vi "RearrangeFrameByNames__slk_mt.vi"(8 "error in (no error)":errorcluster, 10 "frame names":string[](array[string]), 11 "case model in":refnum<class "CaseModel__slk_mt.lvclass">) -> (0 "error out":errorcluster, 3 "case model out":refnum<class "CaseModel__slk_mt.lvclass">)   [LabVIEW 2012, in "Lazyboots Menu Tool.lvlib" / "CaseModel__slk_mt.lvclass"]
doc: "Rearranges frame by specified names array."
uses:
  CaseModel__slk_mt.lvclass
panel:
  # "RearrangeFrameByNames__slk_mt.vi\nRearranges frame by specified names array.\n\nNOTICE -- YOU MUST LEAVE THIS NOTICE IN PLACE.\n\nCopyright (c) 2011, LIANG LIU Shawn.Liu.cn@gmail.com\nAll rights reserved.\n\nRedistribution and use in source and binary forms, with or without modification, are permitted provided that the following conditions are met:\n-Redistributions of source code must retain the above copyright notice, this list of conditions and the following disclaimer.\n-Redistributions in binary form must reproduce the above copyright notice, this list of conditions and the following disclaimer in the documentation and/or other materials provided with the distribution.\n-Neither the name of the eLp nor the names of its contributors may be used to endorse or promote products derived from this software without specific prior written permission.\n\nTHIS SOFTWARE IS PROVIDED BY THE COPYRIGHT HOLDERS AND CONTRIBUTORS \"AS IS\" AND ANY EXPRESS OR IMPLIED WARRANTIES, INCLUDING, BUT NOT LIMITED TO, THE IMPLIED WARRANTIES OF MERCHANTABILITY AND FITNESS FOR A PARTICULAR PURPOSE ARE DISCLAIMED. IN NO EVENT SHALL THE COPYRIGHT HOLDER OR CONTRIBUTORS BE LIABLE FOR ANY DIRECT, INDIRECT, INCIDENTAL, SPECIAL, EXEMPLARY, OR CONSEQUENTIAL DAMAGES (INCLUDING, BUT NOT LIMITED TO, PROCUREMENT OF SUBSTITUTE GOODS OR SERVICES; LOSS OF USE, DATA, OR PROFITS; OR BUSINESS INTERRUPTION) HOWEVER CAUSED AND ON ANY THEORY OF LIABILITY, WHETHER IN CONTRACT, STRICT LIABILITY, OR TORT (INCLUDING NEGLIGENCE OR OTHERWISE) ARISING IN ANY WAY OUT OF THE USE OF THIS SOFTWARE, EVEN IF ADVISED OF THE POSSIBILITY OF SUCH DAMAGE."
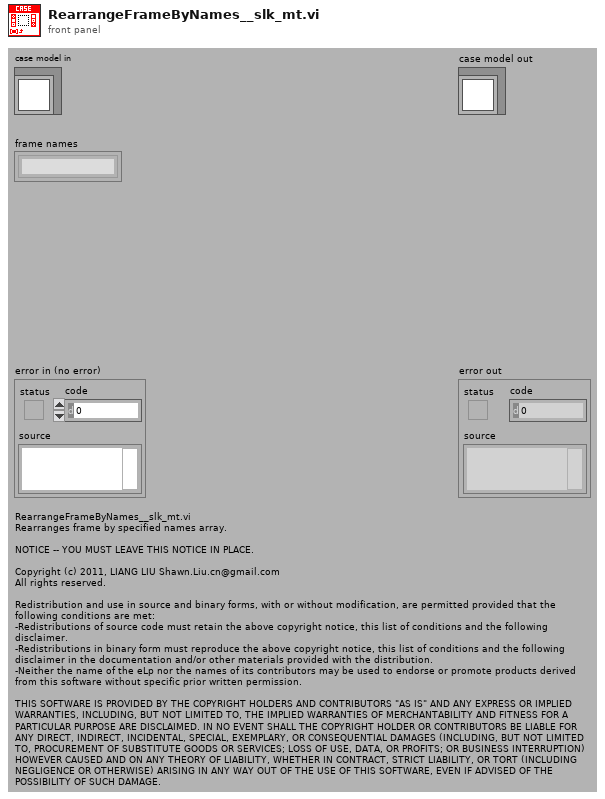
[diagram p1: front panel]
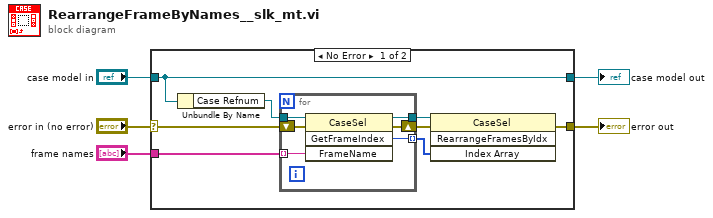
[diagram p0: block diagram]
diagram:
  n1 = case shown="No Error" "error in (no error)" {
    selector: "error in (no error)" -> [w6 w21]
    tunnel: [w9 w21] -> w4
    tunnel: [w8 w20] -> w2
    tunnel: "case model in" -> [w8 w20]
    tunnel: "frame names" -> [w7 _]
    frame No Error {
      n2 = Unbundle By Name(w8) -> ("Case Refnum"=w13:refnum<vi>)
      n3 = for {
        tunnel: w13 -> [w19]
        tunnel: [w18] -> w12
        shift-right: [w17] -> w11
        shift-left: w6 -> [w16]
        tunnel: w7 -> [w15] mode=indexing
        tunnel: [w14] -> w10 mode=indexing
        n4 = invoke class="CaseSel" method="GetFrameIndex"(reference=w19, error in=w16, "FrameName"=w15) -> (reference out=w18:refnum<vi>, error out=w17:errorcluster, "GetFrameIndex"=w14:i32)  [unwired: 1 in, 1 out]
      }
      n5 = invoke class="CaseSel" method="RearrangeFramesByIdx"(reference=w12, error in=w11, "Index Array"=w10) -> (error out=w9:errorcluster)  [unwired: 1 in, 3 out]
    }
    frame Error {
    }
  }
  "error out" <- w4
  "case model out" <- w2
